vi "Initialize-object.vi"(8 "error in (no error)":errorcluster, 10 "VI Reference":refnum<vi>) -> (0 "error out":errorcluster, 3 "Reference out":T1)   [LabVIEW 2013, in "HardwareCharacterization.lvlib" / "HC-ScanParser.lvclass"]
uses:
  HC-ScanParser.lvclass
  Object-reference.ctl
  Laser-properties.ctl
  Field-properties.ctl
  HC-ScanParser.lvclass/HC-ScanParser.ctl
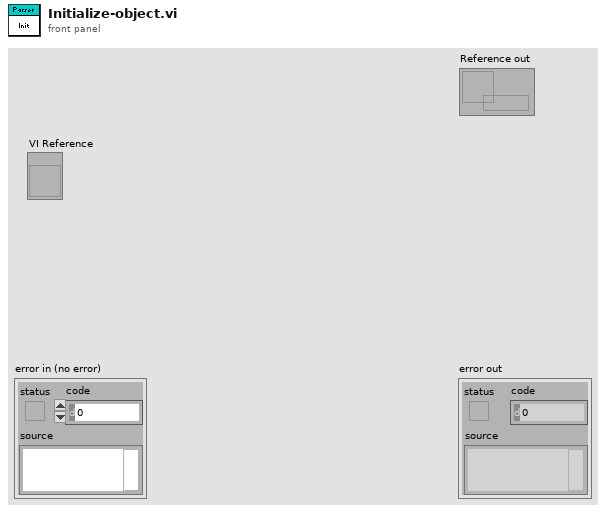
[diagram p1: front panel]
types:
  T1 = typedef "HardwareCharacterization.lvlib/HC-ScanParser.lvclass/Object-reference.ctl" = refnum<data-value>
  T2 = typedef "HardwareCharacterization.lvlib/HC-ScanParser.lvclass/Field-properties.ctl" = cluster{"Layer height":dbl, "MaximumFieldWidth":dbl, "MaximumFieldHeight":dbl, "MaximumFieldRadius":dbl, "MaxAcceleration":dbl, "MaxMarkSpeed":dbl, "MaxJumpSpeed":dbl}
  T3 = typedef "HardwareCharacterization.lvlib/HC-ScanParser.lvclass/Laser-properties.ctl" = cluster{"MaximumLaserPower":dbl, "Power curve":cluster{"Watt":dbl[], "Bits":u8[]}, "Rise time":i64, "Fall time":i64}
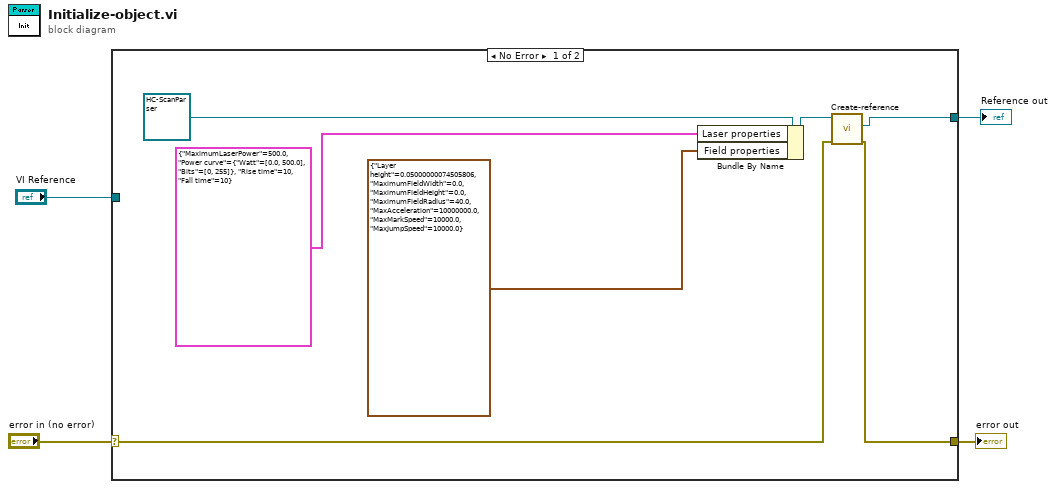
[diagram p0: block diagram]
diagram:
  n1 = case shown="No Error" "error in (no error)" {
    selector: "error in (no error)" -> [w11 w12]
    tunnel: [w9 w12] -> w3
    tunnel: "VI Reference" -> [_ _]
    tunnel: [w8 _] -> w1
    frame No Error {
      n2 = Bundle By Name(cluster=refnum<class "HC-ScanParser.lvclass"> refnum ("Panes.lvclass"), "Laser properties"=T3 {"MaximumLaserPower"=500.0, "Power curve"={"Watt"=[0.0, 500.0], "Bits"=[0, 255]}, "Rise time"=10, "Fall time"=10}, "Field properties"=T2 {"Layer height"=0.05000000074505806, "MaximumFieldWidth"=0.0, "MaximumFieldHeight"=0.0, "MaximumFieldRadius"=40.0, "MaxAcceleration"=10000000.0, "MaxMarkSpeed"=10000.0, "MaxJumpSpeed"=10000.0}) -> (w7:refnum<class "HC-ScanParser.lvclass">)
      n3 = call "Create-reference.vi"("error in (no error)"=w11, "Object in"=w7) -> ("error out"=w9:errorcluster, "Object reference"=w8:T1)  [unwired: 7 in, 1 out]
    }
    frame Error {
    }
  }
  "error out" <- w3
  "Reference out" <- w1
